vi "C_P_FACT.vi"() -> ()   [LabVIEW 2026]
panel:
  in  "Numeric 6":dbl
  in  "Numeric 5":dbl
  in  "Numeric 4":dbl
  out "Numeric 3":dbl
  in  "Numeric 2":i32
  in  "Numeric":dbl
  out "o/p":dbl
  in  "constant":dbl
  in  "range of odd nums":dbl
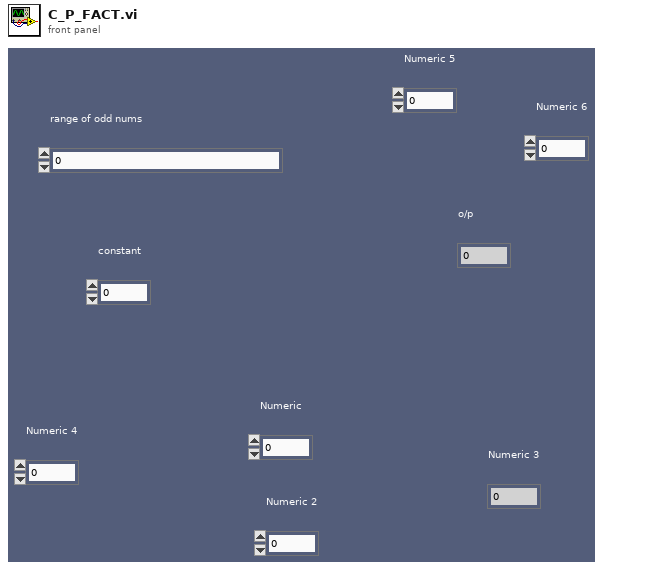
[diagram p1: front panel]
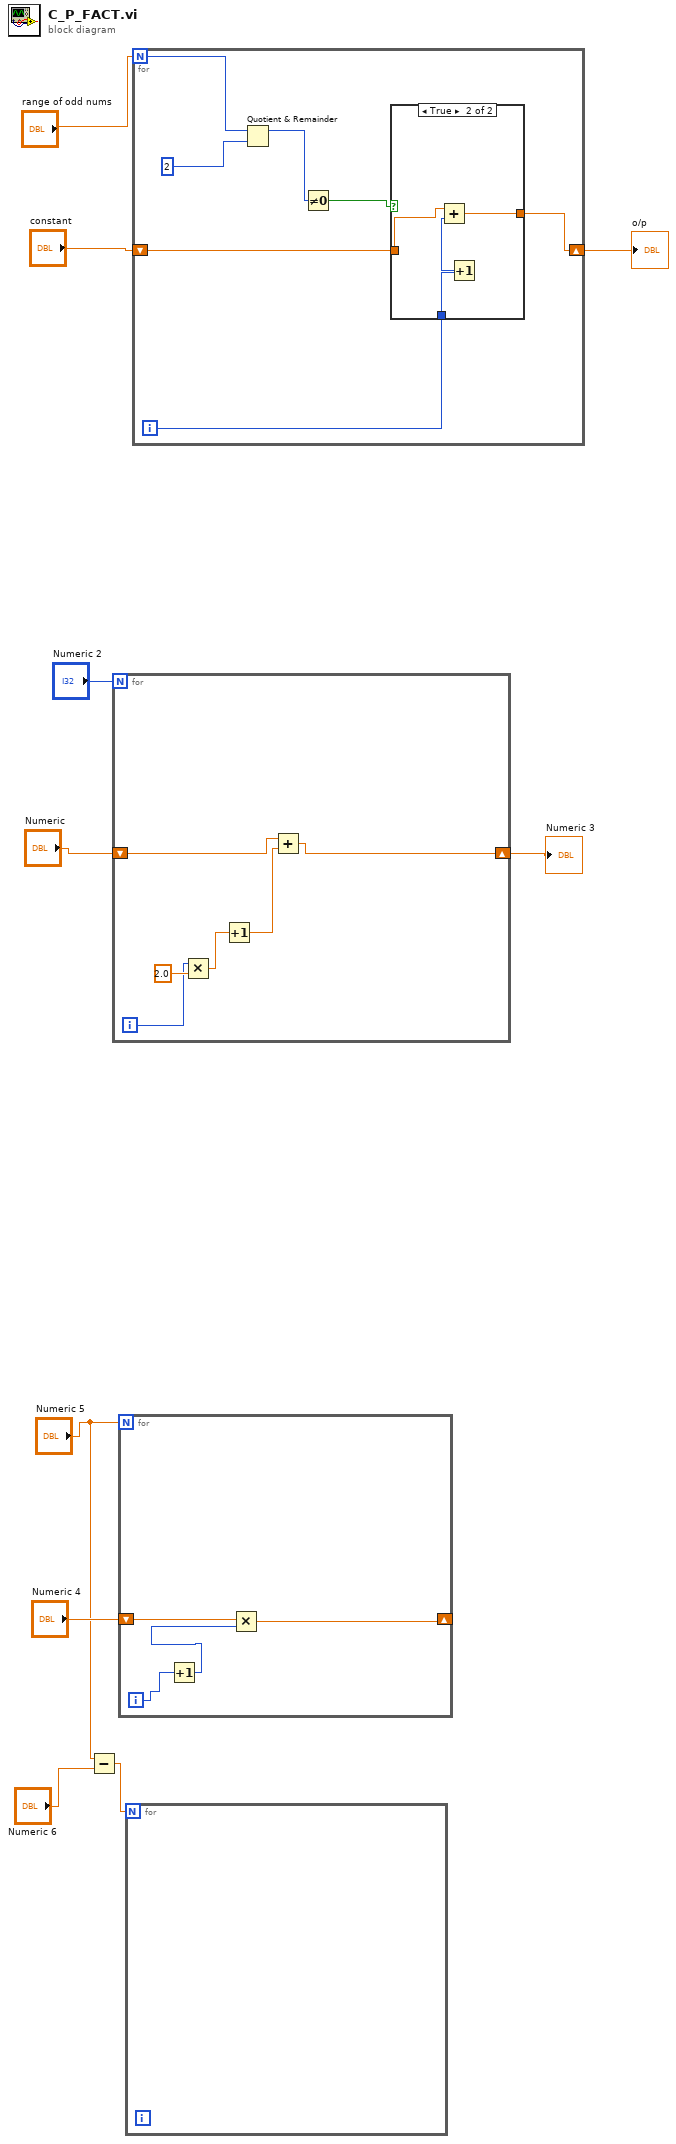
[diagram p0: block diagram]
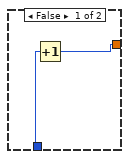
[diagram p2: hidden frame]
diagram:
  n1 = Subtract(x="Numeric 5", y="Numeric 6") -> (x-y=w1:dbl)
  n2 = for {
    N: "Numeric 2" -> [_]
    shift-right: [w12] -> w5
    shift-left: "Numeric" -> [w14]
    i -> [w11]
    n3 = Multiply(x=w11, y=2.0) -> (x*y=w15:dbl)
    n4 = Increment(x=w15) -> (x+1=w13:dbl)
    n5 = Add(x=w14, y=w13) -> (x+y=w12:dbl)
  }
  "Numeric 3" <- w5
  n6 = for {
    N: "Numeric 5" -> [_]
    shift-right: [w19] -> _
    shift-left: "Numeric 4" -> [w20]
    i -> [w18]
    n7 = Increment(x=w18) -> (x+1=w17:i32)
    n8 = Multiply(x=w20, y=w17) -> (x*y=w19:dbl)
  }
  n9 = for {
    N: w1 -> [_]
  }
  n10 = for {
    N: "range of odd nums" -> [w27]
    shift-right: [w21] -> w8
    shift-left: "constant" -> [w23]
    i -> [w22]
    n11 = Quotient & Remainder(x=w27, y=2) -> (x-y*floor(x/y)=w25:i32)  [unwired: 1 out]
    n12 = Not Equal To 0?(x=w25) -> (x != 0?=w24:bool)
    n13 = case shown="True" w24 {
      tunnel: w23 -> [_ w33]
      tunnel: w22 -> [w29 w30]
      tunnel: [w28 w32] -> w21
      frame False {
        n14 = Increment(x=w29) -> (x+1=w28:i32)
      }
      frame True {
        n15 = Increment(x=w30) -> (x+1=w31:i32)
        n16 = Add(x=w33, y=w31) -> (x+y=w32:dbl)
      }
    }
  }
  "o/p" <- w8
